vi "Add Default Value Tree Info.vi"(10 "Default Digital Values":bool[](array[boolean]), 11 "Default Analog Values":dbl[](array[numeric])) -> (1 "Tree Data":T1[](array[typedef]) {"Data Type" items=["Tree Parent"=-1, "Numeric"=0, "String"=1, "Boolean"=2, "Enum"=3]}, 2 "Tags":string[](array[string]), 3 "Tree Items":T3(array[cluster]))   [LabVIEW 2020, in "Sequencer with Output Values.lvlib" / "Sequencer with Output Values.lvclass"]
uses:
  Sequencer with Output Values.lvclass
  Tree Item Settings.ctl
  Data Type.ctl
  Global Tree Data.vi
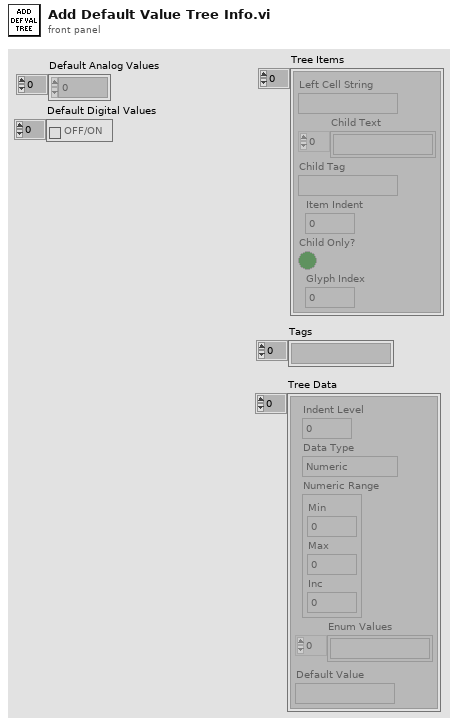
[diagram p1: front panel]
types:
  T1 = typedef "Sequencer with Output Values.lvlib/Sequencer with Output Values.lvclass/Tree Item Settings.ctl" = cluster{"Indent Level":i32, "Data Type":T2, "Numeric Range":cluster{"Min":dbl, "Max":dbl, "Inc":dbl}, "Enum Values":string[], "Default Value":string}
  T2 = typedef "Sequencer with Output Values.lvlib/Sequencer with Output Values.lvclass/Data Type.ctl" = i16
  T3 = cluster{"Left Cell String":string, "Child Text":string[], "Child Tag":string, "Item Indent":i32, "Child Only?":bool, "Glyph Index":i32}[]
  T4 = cluster{"Left Cell String":string, "Child Text":string[], "Child Tag":string, "Item Indent":i32, "Child Only?":bool, "Glyph Index":i32}
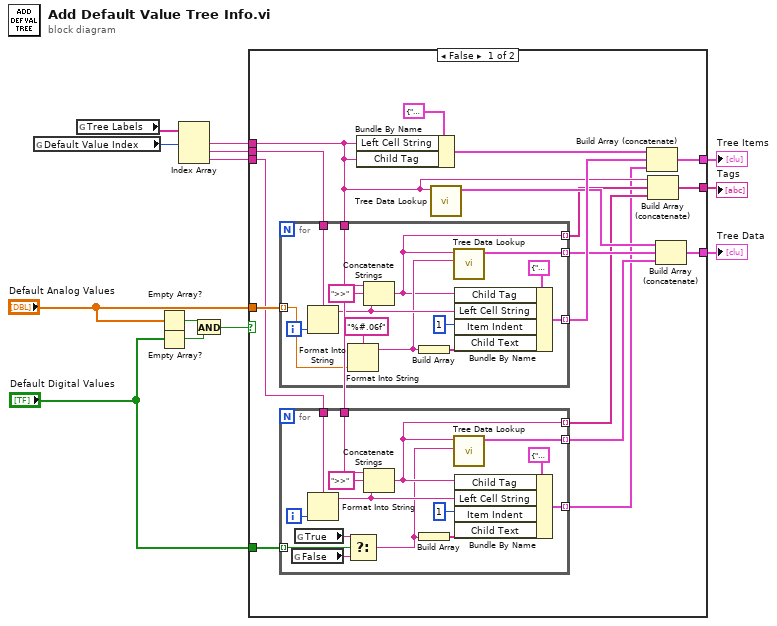
[diagram p0: block diagram]
diagram:
  n1 = global read "Global Tree Data.vi" "Default Value Index"() -> (w11:i32)
  n2 = global read "Global Tree Data.vi" "Tree Labels"() -> (w12:string[])
  n3 = Empty Array?(array="Default Analog Values") -> (empty?=w8:bool)
  n4 = Empty Array?(array="Default Digital Values") -> (empty?=w7:bool)
  n5 = Index Array(array=w12, index #1=w11) -> (element #1=w10:string, element #2=w9:string, element #3=w5:string)  [unwired: 2 in]
  n6 = And(x=w8, y=w7) -> (x .and. y?=w13:bool)
  n7 = case shown="False" w13 {
    tunnel: w10 -> [w22 _]
    tunnel: w9 -> [w29 _]
    tunnel: "Default Analog Values" -> [w28 _]
    tunnel: w5 -> [w21 _]
    tunnel: "Default Digital Values" -> [w20 _]
    tunnel: [w16 _] -> w3
    tunnel: [w15 _] -> w2
    tunnel: [w14 _] -> w1
    frame False {
      n8 = for {
        tunnel: w29 -> [w58]
        tunnel: w22 -> [w55]
        tunnel: w28 -> [w52] mode=indexing
        tunnel: [w49] -> w26 mode=indexing
        tunnel: [w47] -> w25 mode=indexing
        tunnel: [w46] -> w23 mode=indexing
        i -> [w57]
        n9 = Format Into String(format string=w58, w57) -> (resulting string=w54:string)  [unwired: 2 in, 1 out]
        n10 = Format Into String(format string="%#.06f", w52) -> (resulting string=w48:string)  [unwired: 2 in, 1 out]
        n11 = Concatenate Strings(w55, ">>" ("string"), w54) -> (w46:string)
        n12 = Build Array(w48) -> (w50:string[])
        n13 = call "Tree Data Lookup.vi"("Value"=w48, "Key"=w46) -> ("Tree Data"=w47:T1)  [unwired: 9 in]
        n14 = Bundle By Name(cluster=T4 {"Left Cell String"="", "Child Text"=[], "Child Tag"="", "Item Indent"=0, "Child Only?"=FALSE, "Glyph Index"=0} ("Item"), "Child Tag"=w46, "Left Cell String"=w54, "Item Indent"=1, "Child Text"=w50) -> (w49:T4)
      }
      n15 = for {
        tunnel: w21 -> [w44]
        tunnel: w22 -> [w41]
        tunnel: w20 -> [w34] mode=indexing
        tunnel: [w37] -> w17 mode=indexing
        tunnel: [w36] -> w18 mode=indexing
        tunnel: [w35] -> w19 mode=indexing
        i -> [w43]
        n16 = global read "Global Tree Data.vi" "False"() -> (w32:string)
        n17 = global read "Global Tree Data.vi" "True"() -> (w33:string)
        n18 = Format Into String(format string=w44, w43) -> (resulting string=w40:string)  [unwired: 2 in, 1 out]
        n19 = Select(t=w33, s=w34, f=w32) -> (s? t:f=w31:string)
        n20 = Concatenate Strings(w41, ">>" ("string"), w40) -> (w35:string)
        n21 = Build Array(w31) -> (w38:string[])
        n22 = call "Tree Data Lookup.vi"("Value"=w31, "Key"=w35) -> ("Tree Data"=w36:T1)  [unwired: 9 in]
        n23 = Bundle By Name(cluster=T4 {"Left Cell String"="", "Child Text"=[], "Child Tag"="", "Item Indent"=0, "Child Only?"=FALSE, "Glyph Index"=0} ("Item"), "Child Tag"=w35, "Left Cell String"=w40, "Item Indent"=1, "Child Text"=w38) -> (w37:T4)
      }
      n24 = Bundle By Name(cluster=T4 {"Left Cell String"="", "Child Text"=[], "Child Tag"="", "Item Indent"=0, "Child Only?"=FALSE, "Glyph Index"=0} ("Item"), "Left Cell String"=w22, "Child Tag"=w22) -> (w27:T4)
      n25 = call "Tree Data Lookup.vi"("Key"=w22) -> ("Tree Data"=w24:T1)  [unwired: 10 in]
      n26 = Build Array (concatenate)(w27, w26, w17) -> (w16:T3)
      n27 = Build Array (concatenate)(w22, w23, w19) -> (w15:string[])
      n28 = Build Array (concatenate)(w24, w25, w18) -> (w14:T1[])
    }
    frame True {
    }
  }
  "Tree Items" <- w3
  "Tags" <- w2
  "Tree Data" <- w1
